vi "SlowLogger_LogThisSlowly.vi"(6 "Over ride time stamp (default do not wire)\nNote: MIDAS history plots cannot write data into the past":timestamp, 8 "error in (no error)":errorcluster, 10 "Array":dbl[](array[numeric]), 11 "SlowLogger in":refnum<class "SlowLogger.lvclass">) -> (0 "error out":errorcluster, 1 "Dt satisfied (data logged)":bool=TRUE, 2 "Dt (s)":dbl, 3 "SlowLogger out":refnum<class "SlowLogger.lvclass">)   [LabVIEW 2018, in "feGEM DataPacker.lvlib" / "SlowLogger.lvclass"]
uses:
  SlowLogger.lvclass
  SlowLogger.lvclass/SlowLogger.ctl
  f93abad2-5217-430f-97d3-b2f2641e9ea3.vi
  f93abad2-5217-430f-97d3-b2f2641e9ea3.vi/267d003a-726b-4b2a-b061-444b575c69a8.vi
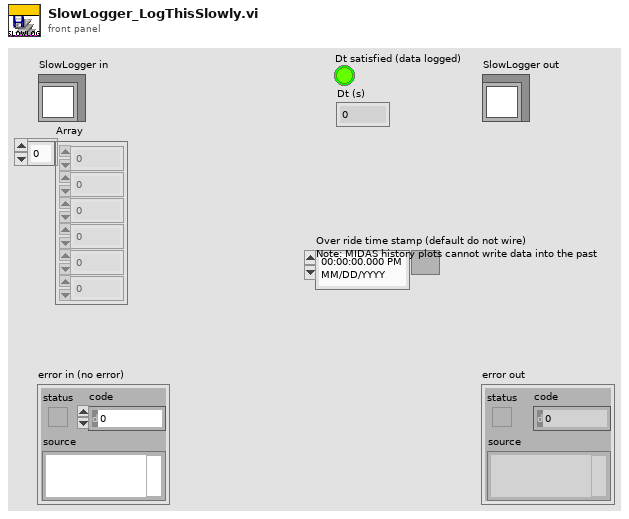
[diagram p1: front panel]
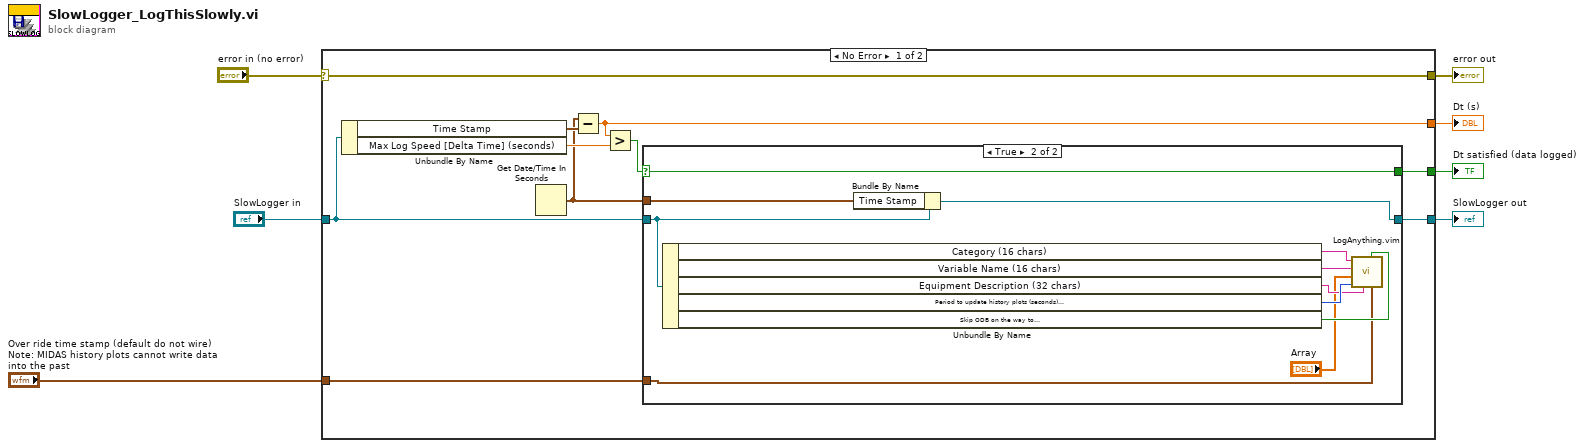
[diagram p0: block diagram]
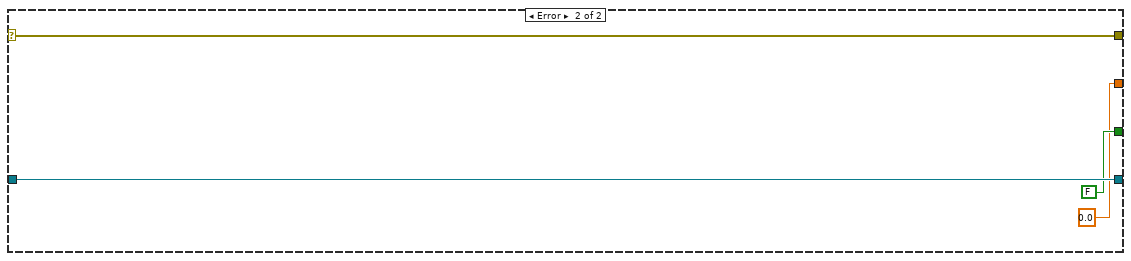
[diagram p3: hidden frame]
diagram:
  n1 = case shown="No Error" "error in (no error)" {
    selector: "error in (no error)" -> [w17 w33]
    tunnel: [w17 w33] -> w6
    tunnel: [w10 w34] -> w4
    tunnel: "SlowLogger in" -> [w14 w34]
    tunnel: [w13 FALSE] -> w3
    tunnel: [w12 0.0] -> w2
    tunnel: "Over ride time stamp (default do not wire)\nNote: MIDAS history plots cannot write data into the past" -> [w8 _]
    frame No Error {
      n2 = Unbundle By Name(w14) -> ("Time Stamp"=w11:timestamp, "Max Log Speed [Delta Time] (seconds)"=w16:dbl)
      n3 = Get Date/Time In Seconds() -> (seconds since 1Jan1904=w9:timestamp)
      n4 = Subtract(x=w9, y=w11) -> (x-y=w12:dbl)
      n5 = Greater?(x=w12, y=w16) -> (0:w15:bool)
      n6 = case shown="True" w15 {
        selector: w15 -> [w19 w24]
        tunnel: w14 -> [w18 w23]
        tunnel: [w19 w24] -> w13
        tunnel: w9 -> [_ w22]
        tunnel: [w18 w21] -> w10
        tunnel: w8 -> [_ w20]
        frame False {
        }
        frame True {
          n7 = Unbundle By Name(w23) -> ("Category (16 chars)"=w25:string, "Variable Name (16 chars)"=w26:string, "Equipment Description (32 chars)"=w28:string, "Period to update history plots (seconds)\nUnset (65535) = Use MIDAS default in ODB\n0 = Record but do not put in histories"=w30:u16, "Skip ODB on the way to \nhistories (fast, but no ALARMS possible)"=w29:bool)
          n8 = Bundle By Name(cluster=w23, "Time Stamp"=w22) -> (w21:refnum<class "SlowLogger.lvclass">)
          n9 = call "LogAnything.vim"("Over ride time stamp (default do not wire)\nNote: MIDAS history plots cannot write data into the past"=w20, "Skip ODB on the way to \nhistories (fast, but no ALARMS possible)"=w29, "Equipment description (32 chars)"=w28, "Period to update history plots (seconds)\nUnset (65535) = Use MIDAS default in ODB\n0 = Record but do not put in histories"=w30, "Array"="Array", "Variable Name"=w26, "Category"=w25) -> ()  [unwired: 3 in, 2 out]
        }
      }
    }
    frame Error {
    }
  }
  "error out" <- w6
  "SlowLogger out" <- w4
  "Dt satisfied (data logged)" <- w3
  "Dt (s)" <- w2
